vi "FRCts20_Backend_Test_RequestRoot_POST.vi"(8 "error in (no error)":errorcluster, 10 "Description":string, 11 "Team Index":u32) -> (0 "error out":errorcluster, 1 "Time (ms)":u32, 2 "Status":string, 3 "Request Out":T1, 5 "Success":bool)   [LabVIEW 2013, in "FRCts20_Backend_TestCode.lvlib"]
uses:
  FRCts20_Backend_TestCode.lvlib
  FRCts20_Backend_API/FRCts20_Backend_API_RequestRoot.ctl
  FRCts20_Backend_API/FRCts20_Backend_API_Status.ctl
  FRCts20_Backend_API/FRCts20_Backend_API_Command_RequestRoot.ctl
  FRCts20_Backend_API/FRCts20_Backend_API_RequestRoot.vi
  FRCts20_Backend_API/FRCts20_Backend_API.lvlib
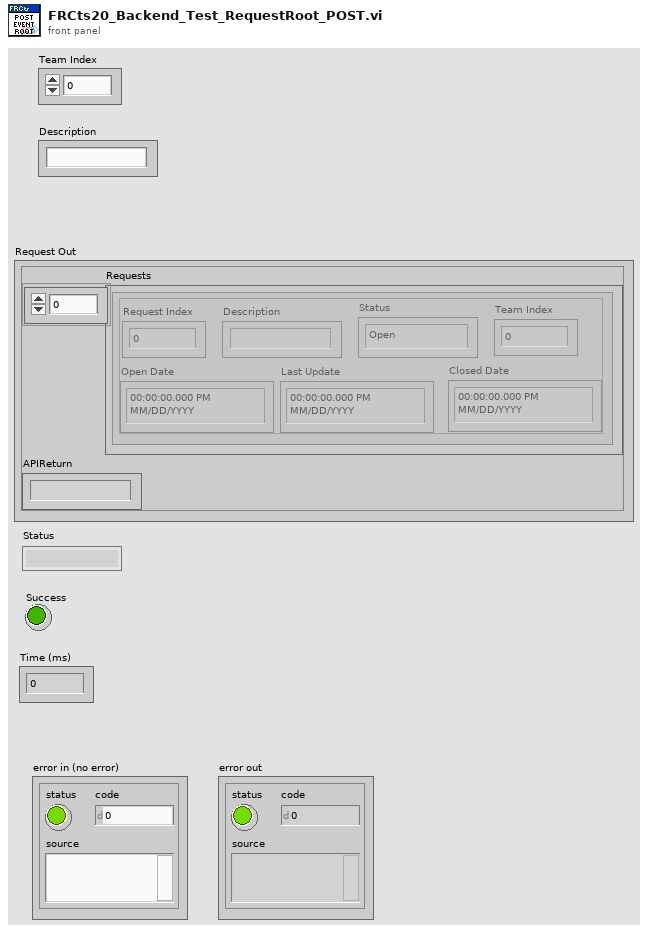
[diagram p1: front panel]
types:
  T1 = typedef "FRCts20_Backend_API.lvlib/FRCts20_Backend_API_RequestRoot.ctl" = cluster{"Requests":cluster{"Request Index":u32, "Description":string, "Status":T2, "Open Date":timestamp, "Last Update":timestamp, "Closed Date":timestamp, "Team Index":u32}[], "APIReturn":string}
  T2 = typedef "FRCts20_Backend_API.lvlib/FRCts20_Backend_API_Status.ctl" = enum16{"Open", "In Work", "Closed"}
  T3 = typedef "FRCts20_Backend_API.lvlib/FRCts20_Backend_API_Command_RequestRoot.ctl" = string
  T4 = cluster{"Request Index":u32, "Description":string, "Status":T2, "Open Date":timestamp, "Last Update":timestamp, "Closed Date":timestamp, "Team Index":u32}[]
  T5 = cluster{"Request Index":u32, "Description":string, "Status":T2, "Open Date":timestamp, "Last Update":timestamp, "Closed Date":timestamp, "Team Index":u32}
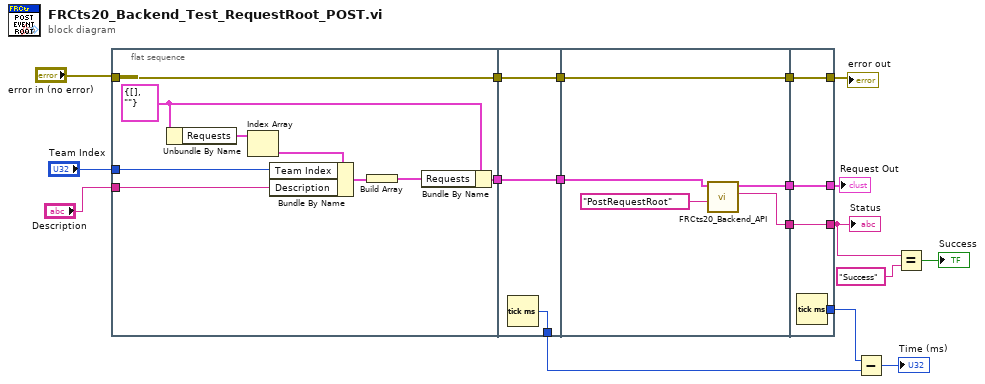
[diagram p0: block diagram]
diagram:
  n1 = flat-sequence {
    tunnel: "error in (no error)" -> [w27]
    tunnel: [w27] -> w18
    tunnel: "Team Index" -> [w24]
    tunnel: "Description" -> [w23]
    tunnel: [w19] -> w1
    tunnel: [w30] -> w7
    tunnel: [w29] -> w17
    tunnel: w18 -> [w29]
    tunnel: [w28] -> w2
    tunnel: w1 -> [w28]
    tunnel: [w35] -> w16
    tunnel: w17 -> [w35]
    tunnel: [w34] -> w15
    tunnel: [w33] -> w14
    tunnel: w2 -> [w31]
    tunnel: [w39] -> w8
    tunnel: [w38] -> w10
    tunnel: w16 -> [w38]
    tunnel: [w37] -> w5
    tunnel: w15 -> [w37]
    tunnel: [w36] -> w6
    tunnel: w14 -> [w36]
    frame #0 {
      w21 = T1 {"Requests"=[], "APIReturn"=""} ("Request In")
      n2 = Unbundle By Name(w21) -> ("Requests"=w26:T4)
      n3 = Index Array(array=w26) -> (element=w25:T5)  [unwired: 1 in]
      n4 = Bundle By Name(cluster=w25, "Team Index"=w24, "Description"=w23) -> (w22:T5)
      n5 = Build Array(w22) -> (w20:T4)
      n6 = Bundle By Name(cluster=w21, "Requests"=w20) -> (w19:T1)
    }
    frame #1 {
      n7 = Tick Count (ms)() -> (millisecond timer value=w30:u32)
    }
    frame #2 {
      n8 = call-poly "FRCts20_Backend_API.vi"("Message"=T3 "PostRequestRoot", "Request In"=w31) -> ("Status"=w33:string, "Request Out"=w34:T1)  [unwired: 7 in, 1 out]
    }
    frame #3 {
      n9 = Tick Count (ms)() -> (millisecond timer value=w39:u32)
    }
  }
  n10 = Subtract(x=w8, y=w7) -> (x-y=→"Time (ms)":u32)
  n11 = Equal?(x=w6, y="Success") -> (x = y?=→"Success":bool)
  "Status" <- w6
  "error out" <- w10
  "Request Out" <- w5
